vi "Convert Controls to Arrays.vi"(9 "ConPane Only?":bool, 11 "Ctl Properties":T1[](array[typedef])) -> (3 "Control Array":string[][](array[string]))   [LabVIEW 2023, in "VI Properties Editor.lvlib"]
doc: "Converts <B>Ctl Properties</B> to arrays to be displayed to the user."
uses:
  VI Properties Editor.lvlib
  CTLs/Control Properties.ctl
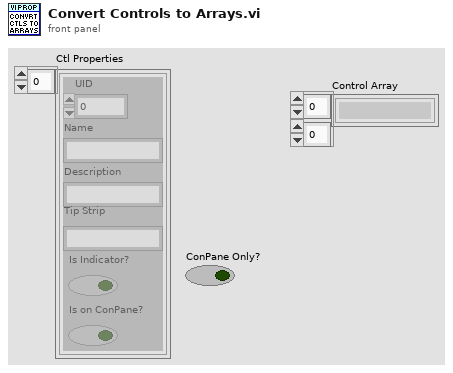
[diagram p1: front panel]
types:
  T1 = typedef "VI Properties Editor.lvlib/Control Properties.ctl" = cluster{"UID":i32, "Name":string, "Description":string, "Tip Strip":string, "Is Indicator?":bool, "Is on ConPane?":bool}
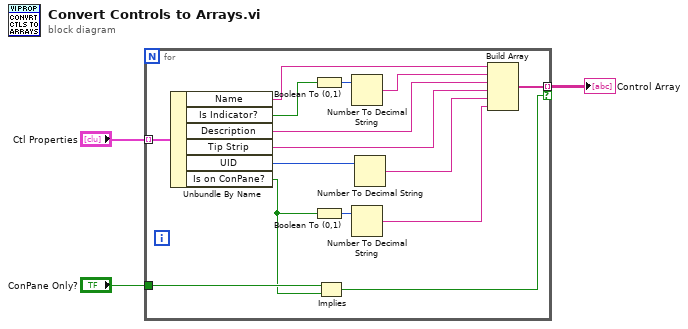
[diagram p0: block diagram]
diagram:
  n1 = for {
    tunnel: [w9] -> w2 mode=indexing if=w7
    tunnel: "Ctl Properties" -> [w18] mode=indexing
    tunnel: "ConPane Only?" -> [w8]
    n2 = Unbundle By Name(w18) -> ("Name"=w17:string, "Is Indicator?"=w15:bool, "Description"=w13:string, "Tip Strip"=w12:string, "UID"=w11:i32, "Is on ConPane?"=w5:bool)
    n3 = Boolean To (0,1)(Boolean=w15) -> (0, 1=w16:i16)
    n4 = Boolean To (0,1)(Boolean=w5) -> (0, 1=w6:i16)
    n5 = Implies(1:w5, 2:w8) -> (0:w7:bool)
    n6 = Number To Decimal String(number=w16) -> (decimal integer string=w14:string)  [unwired: 1 in]
    n7 = Number To Decimal String(number=w6) -> (decimal integer string=w4:string)  [unwired: 1 in]
    n8 = Number To Decimal String(number=w11) -> (decimal integer string=w10:string)  [unwired: 1 in]
    n9 = Build Array(w17, w14, w13, w12, w10, w4) -> (w9:string[])
  }
  "Control Array" <- w2
